vi "DAQ_global.vi"() -> ()   [LabVIEW 2013]
panel:
  out "meas_rms":dbl
  in  "meas_freq":dbl
  in  "meas_THD":dbl
  in  "meas_peak":dbl
  in  "meas_amp":dbl
  in  "ADC_rate":dbl
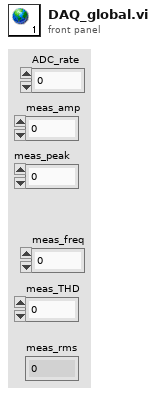
[diagram p1: front panel]
diagram:
